vi "SP Read Single.vi"(8 "error in":errorcluster, 9 "Channel Index":i32=1, 11 "Power Setpoint in":refnum<class "Power Setpoint.lvclass">) -> (0 "error out":errorcluster, 1 "Changed or First Call?":bool, 2 "Power SP":dbl, 3 "Power Setpoint out":refnum<class "Power Setpoint.lvclass">)   [LabVIEW 2023, in "Power Setpoint.lvclass"]
uses:
  Power Setpoint.lvclass
  Parents/Setpoint/Setpoint.lvclass
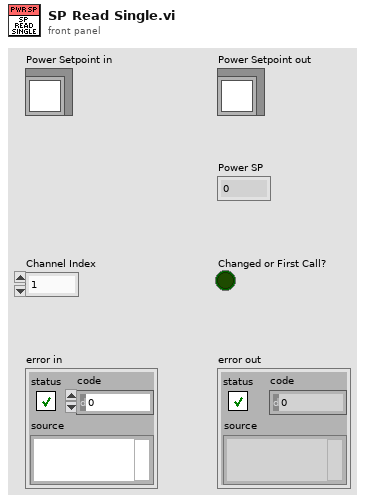
[diagram p1: front panel]
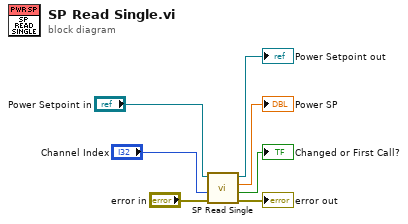
[diagram p0: block diagram]
diagram:
  n1 = call-parent "SP Read Single.vi"("error in"="error in", "Channel Index"="Channel Index", "Setpoint in"="Power Setpoint in") -> ("error out"=→"error out":errorcluster, "Changed or First Call?"=→"Changed or First Call?":bool, "Current SP"=→"Power SP":dbl, "Setpoint out"=→"Power Setpoint out":refnum<class "Power Setpoint.lvclass">)  [unwired: 5 in]
